vi "Empty_Complete.vi"(11 "input cluster":T1={"L16 Linear Actuator"="", "XE 1000 Pump"="", "Camera1"="", "Camera2"="", "Camera1_IMG"=refnum, "Camera2_IMG"=refnum, "Img_Capt"=FALSE, "Actuator"=FALSE, "Pump"=FALSE, "Cam 1"=FALSE, "Cam 2"=FALSE, "Empty_Refill"=FALSE, "Crop"=FALSE, "Light intensity"=100, "Exposure Time"=1000.0, "Sample Name"="Test Sample", "Operator"="MRJ", "Calibration 1"=path "C:/Users/au540322/Desktop/IHS_Project/images/Debris/Debris_0/Debris_0_2019_06_01-23-32-49-686.PNG", "Calibration 2"=path "C:/Users/au540322/Desktop/IHS_Project/images/Debris/Debris_0/Debris_0_2019_06_01-23-32-49-686.PNG", "Framerate"=1, "Timeout Sample"=0, "Collection date"="MRJ", "Sample size threshold"=1, "Empty start"=1, "Command"="MRJ", "Calibration Image 1"=refnum, "Calibration Image 2"=refnum, "Original Image 1"=refnum, "Original Image 2"=refnum, "Processing Image 1"=refnum, "Processing Image 2"=refnum, "Object Image 1"=refnum, "Object Image 2"=refnum, "Cam 1 - save queue"=refnum, "Cam 2 - save queue"=refnum, "Station"="", "Species Name"="", "Other Notes"="", "Aperture"=enum."Item 0", "Image Process Queue Size"=500, "Image Save Queue Size"=500, "Overload threshold"=500, "Max Framerate"=100, "Blue Plane Image"=refnum, "Subtract Image"=refnum, "Binary Image 1"=refnum, "ROI mask allocation"=refnum, "Rectangle 1"={"Left"=0, "Top"=0, "Right"=0, "Bottom"=0, "Rotation"=0.0}, "Rectangle 2"={"Left"=0, "Top"=0, "Right"=0, "Bottom"=0, "Rotation"=0.0}, "Binary Image 2"=refnum, "Detection Region %"=0.0, "Cam 1 queue"=refnum, "Cam 2 queue"=refnum, "Detect image 1"=refnum, "Detect image 2"=refnum, "Detect 1"=path "C:/Users/au540322/Desktop/IHS_Project/images/Debris/Debris_0/Debris_0_2019_06_01-23-32-49-686.PNG", "Detect 2"=path "C:/Users/au540322/Desktop/IHS_Project/images/Debris/Debris_0/Debris_0_2019_06_01-23-32-49-686.PNG", "Max large object threshold"=0, "Open(T)/Close(F)"=FALSE} {"Rectangle 2"."Rotation" format="%.2f"; "Rectangle 2"."Left" scale=0.0..1024.0; "Rectangle 2"."Right" scale=0.0..1024.0; "Rectangle 1"."Rotation" format="%.2f"; "Rectangle 1"."Left" scale=0.0..1024.0; "Rectangle 1"."Right" scale=0.0..1024.0; "Max Framerate" min=1; "Overload threshold" min=1; "Image Save Queue Size" min=1; "Image Process Queue Size" min=1; "Empty start" min=1; "Sample size threshold" min=1; "Framerate" min=1; "Light intensity" scale=0.0..100.0}) -> (0 "Next State":T5=enum."Pump Cycle", 3 "output cluster":T1={"L16 Linear Actuator"="", "XE 1000 Pump"="", "Camera1"="", "Camera2"="", "Camera1_IMG"=refnum, "Camera2_IMG"=refnum, "Img_Capt"=FALSE, "Actuator"=FALSE, "Pump"=FALSE, "Cam 1"=FALSE, "Cam 2"=FALSE, "Empty_Refill"=FALSE, "Crop"=FALSE, "Light intensity"=100, "Exposure Time"=1000.0, "Sample Name"="Test Sample", "Operator"="MRJ", "Calibration 1"=path "C:/Users/au540322/Desktop/IHS_Project/images/Debris/Debris_0/Debris_0_2019_06_01-23-32-49-686.PNG", "Calibration 2"=path "C:/Users/au540322/Desktop/IHS_Project/images/Debris/Debris_0/Debris_0_2019_06_01-23-32-49-686.PNG", "Framerate"=100, "Timeout Sample"=200, "Collection date"="", "Sample size threshold"=500, "Empty start"=1, "Command"="", "Calibration Image 1"=refnum, "Calibration Image 2"=refnum, "Original Image 1"=refnum, "Original Image 2"=refnum, "Processing Image 1"=refnum, "Processing Image 2"=refnum, "Object Image 1"=refnum, "Object Image 2"=refnum, "Cam 1 - save queue"=refnum, "Cam 2 - save queue"=refnum, "Station"="", "Species Name"="", "Other Notes"="", "Aperture"=enum."Item 0", "Image Process Queue Size"=500, "Image Save Queue Size"=500, "Overload threshold"=500, "Max Framerate"=100, "Blue Plane Image"=refnum, "Subtract Image"=refnum, "Binary Image 1"=refnum, "ROI mask allocation"=refnum, "Rectangle 1"={"Left"=0, "Top"=0, "Right"=0, "Bottom"=0, "Rotation"=0.0}, "Rectangle 2"={"Left"=0, "Top"=0, "Right"=0, "Bottom"=0, "Rotation"=0.0}, "Binary Image 2"=refnum, "Detection Region %"=0.0, "Cam 1 queue"=refnum, "Cam 2 queue"=refnum, "Detect image 1"=refnum, "Detect image 2"=refnum, "Detect 1"=path "C:/Users/au540322/Desktop/IHS_Project/images/Debris/Debris_0/Debris_0_2019_06_01-23-32-49-686.PNG", "Detect 2"=path "C:/Users/au540322/Desktop/IHS_Project/images/Debris/Debris_0/Debris_0_2019_06_01-23-32-49-686.PNG", "Max large object threshold"=0, "Open(T)/Close(F)"=FALSE} {"Rectangle 2"."Rotation" format="%.2f"; "Rectangle 2"."Left" scale=0.0..1024.0; "Rectangle 2"."Right" scale=0.0..1024.0; "Rectangle 1"."Rotation" format="%.2f"; "Rectangle 1"."Left" scale=0.0..1024.0; "Rectangle 1"."Right" scale=0.0..1024.0; "Max Framerate" min=1; "Overload threshold" min=1; "Image Save Queue Size" min=1; "Image Process Queue Size" min=1; "Empty start" min=1; "Sample size threshold" min=1; "Framerate" min=1; "Light intensity" scale=0.0..100.0})   [LabVIEW 2019]
uses:
  controls/Data.ctl
  <vilib>/userdefined/High Color/IMAQdx.ctl
  <vilib>/vision/Image Controls.llb/IMAQ Image.ctl
  controls/State.ctl
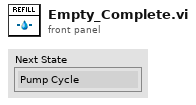
[diagram p1: front panel]
types:
  T1 = typedef "Data.ctl" = cluster{"L16 Linear Actuator":refnum<visa-resource-name>, "XE 1000 Pump":refnum<visa-resource-name>, "Camera1":T2, "Camera2":T2, "Camera1_IMG":T3, "Camera2_IMG":T3, "Img_Capt":bool, "Actuator":bool, "Pump":bool, "Cam 1":bool, "Cam 2":bool, "Empty_Refill":bool, "Crop":bool, "Light intensity":i32, "Exposure Time":dbl, "Sample Name":string, "Operator":string, "Calibration 1":path, "Calibration 2":path, "Framerate":i32, "Timeout Sample":i32, "Collection date":string, "Sample size threshold":i32, "Empty start":u32, "Command":string, "Calibration Image 1":T3, "Calibration Image 2":T3, "Original Image 1":T3, "Original Image 2":T3, "Processing Image 1":T3, "Processing Image 2":T3, "Object Image 1":T3, "Object Image 2":T3, "Cam 1 - save queue":refnum<queue>, "Cam 2 - save queue":refnum<queue>, "Station":string, "Species Name":string, "Other Notes":string, "Aperture":enum32{"Item 0", "Item 1", "Item 2", "Item 3"}, "Image Process Queue Size":i32, "Image Save Queue Size":i32, "Overload threshold":i32, "Max Framerate":i32, "Blue Plane Image":T3, "Subtract Image":T3, "Binary Image 1":T3, "ROI mask allocation":T3, "Rectangle 1":T4, "Rectangle 2":T4, "Binary Image 2":T3, "Detection Region %":dbl, "Cam 1 queue":refnum<queue>, "Cam 2 queue":refnum<queue>, "Detect image 1":T3, "Detect image 2":T3, "Detect 1":path, "Detect 2":path, "Max large object threshold":i32, "Open(T)/Close(F)":bool}
  T2 = typedef "IMAQdx.ctl" = refnum<k21>
  T3 = typedef "IMAQ Image.ctl" = refnum<image>
  T4 = typedef "IMAQ Rectangle" = cluster{"Left":i32, "Top":i32, "Right":i32, "Bottom":i32, "Rotation":dbl}
  T5 = typedef "State.ctl" = enum16{"Initialize", "Wait for Event", "Position", "Valve Signal", "Extra Flush", "Valve Cycle", "Valve Open", "Valve Close", "Pump Command", "Pump Cycle", "Empty System", "Start System", "Connect Systems", "Start Image Capture", "Stop Image Capture", "Calibration Pictures", "Empty and Refill", "Change Light Intensity", "Reconnect", "Exit"}
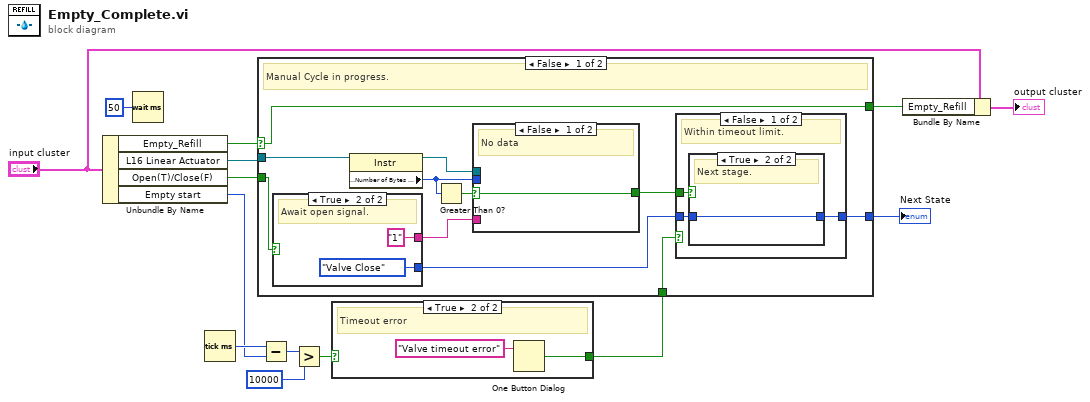
[diagram p0: block diagram]
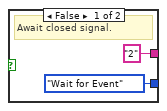
[diagram p3: hidden frame]
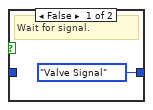
[diagram p4: hidden frame]
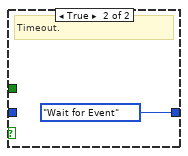
[diagram p5: hidden frame]
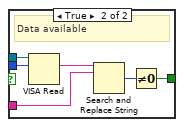
[diagram p6: hidden frame]
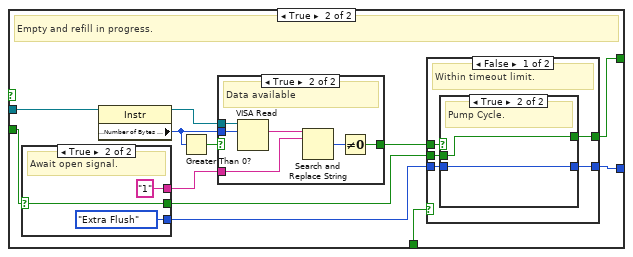
[diagram p7: hidden frame]
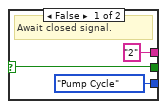
[diagram p8: hidden frame]
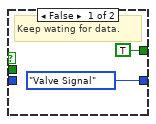
[diagram p9: hidden frame]
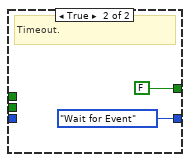
[diagram p10: hidden frame]
diagram:
  n1 = Unbundle By Name("input cluster") -> ("Empty_Refill"=w14:bool, "L16 Linear Actuator"=w13:refnum<visa-resource-name>, "Open(T)/Close(F)"=w1:bool, "Empty start"=w5:u32)
  n2 = Wait (ms)(milliseconds to wait=u32 50) -> ()  [unwired: 1 out]
  n3 = Tick Count (ms)() -> (millisecond timer value=w12:u32)
  n4 = Subtract(x=w12, y=w5) -> (x-y=w11:u32)
  n5 = Greater?(x=w11, y=u32 10000 ("x")) -> (0:w9:bool)
  n6 = case shown="True" w9 {
    selector: w9 -> [w15 _]
    tunnel: [w15 w16] -> w6
    frame False {
      # "Within timeout limit."
    }
    frame True {
      # "Timeout error"
      n7 = One Button Dialog(message="Valve timeout error") -> (true=w16:bool)  [unwired: 1 in]
    }
  }
  n8 = case shown="False" w14 {
    selector: w14 -> [w18 _]
    tunnel: w13 -> [w25 w54]
    tunnel: [w24 w53] -> w7
    tunnel: w6 -> [w23 w52]
    tunnel: [w18 w50] -> w3
    tunnel: w1 -> [w20 w49]
    frame False {
      # "Manual Cycle in progress."
      n9 = case shown="True" w20 {
        tunnel: ["2" ("y") "1" ("y")] -> w21
        tunnel: [State."Wait for Event" ("Next State") State."Valve Close" ("Next State")] -> w19
        frame False {
          # "Await closed signal."
        }
        frame True {
          # "Await open signal."
        }
      }
      n10 = property class="Instr"(reference=w25) -> (reference out=w26:refnum<visa-resource-name>, "Serial Settings:Number of Bytes at Serial Port"=w27:u32)  [unwired: 1 in, 1 out]
      n11 = Greater Than 0?(x=w27) -> (x > 0?=w28:bool)
      n12 = case shown="False" w28 {
        selector: w28 -> [w39 _]
        tunnel: w27 -> [_ w45]
        tunnel: w26 -> [_ w44]
        tunnel: [w39 w43] -> w22
        tunnel: w21 -> [_ w40]
        frame False {
          # "No data"
        }
        frame True {
          # "Data available"
          n13 = VISA Read(VISA resource name=w44, byte count=w45) -> (read buffer=w42:string)  [unwired: 1 in, 3 out]
          n14 = Search and Replace String(input string=w42, search string=w40) -> (number of replacements=w41:i32)  [unwired: 6 in, 3 out]
          n15 = Not Equal To 0?(x=w41) -> (x != 0?=w43:bool)
        }
      }
      n16 = case shown="False" w23 {
        tunnel: [w35 State."Wait for Event" ("Next State")] -> w24
        tunnel: w22 -> [w34 _]
        tunnel: w19 -> [w33 _]
        frame False {
          # "Within timeout limit."
          n17 = case shown="True" w34 {
            tunnel: [State."Valve Signal" ("Next State") w37] -> w35
            tunnel: w33 -> [_ w37]
            frame False {
              # "Wait for signal."
            }
            frame True {
              # "Next stage."
            }
          }
        }
        frame True {
          # "Timeout."
        }
      }
    }
    frame True {
      # "Empty and refill in progress."
      n18 = case shown="True" w49 {
        selector: w49 -> [w58 w61]
        tunnel: ["2" ("y") "1" ("y")] -> w48
        tunnel: [State."Pump Cycle" ("Next State") State."Extra Flush" ("Next State")] -> w47
        tunnel: [w58 w61] -> w46
        frame False {
          # "Await closed signal."
        }
        frame True {
          # "Await open signal."
        }
      }
      n19 = property class="Instr"(reference=w54) -> (reference out=w55:refnum<visa-resource-name>, "Serial Settings:Number of Bytes at Serial Port"=w56:u32)  [unwired: 1 in, 1 out]
      n20 = Greater Than 0?(x=w56) -> (x > 0?=w57:bool)
      n21 = case shown="True" w57 {
        selector: w57 -> [w75 _]
        tunnel: w56 -> [_ w81]
        tunnel: w55 -> [_ w80]
        tunnel: [w75 w79] -> w51
        tunnel: w48 -> [_ w76]
        frame False {
          # "No data"
        }
        frame True {
          # "Data available"
          n22 = VISA Read(VISA resource name=w80, byte count=w81) -> (read buffer=w78:string)  [unwired: 1 in, 3 out]
          n23 = Search and Replace String(input string=w78, search string=w76) -> (number of replacements=w77:i32)  [unwired: 6 in, 3 out]
          n24 = Not Equal To 0?(x=w77) -> (x != 0?=w79:bool)
        }
      }
      n25 = case shown="False" w52 {
        tunnel: [w68 State."Wait for Event" ("Next State")] -> w53
        tunnel: w51 -> [w67 _]
        tunnel: [w66 FALSE] -> w50
        tunnel: w47 -> [w65 _]
        tunnel: w46 -> [w64 _]
        frame False {
          # "Within timeout limit."
          n26 = case shown="True" w67 {
            tunnel: [State."Valve Signal" ("Next State") w72] -> w68
            tunnel: [TRUE w71] -> w66
            tunnel: w65 -> [_ w72]
            tunnel: w64 -> [_ w71]
            frame False {
              # "Keep wating for data."
            }
            frame True {
              # "Pump Cycle."
            }
          }
        }
        frame True {
          # "Timeout."
        }
      }
    }
  }
  "Next State" <- w7
  n27 = Bundle By Name(cluster="input cluster", "Empty_Refill"=w3) -> (→"output cluster":T1)
